vi "Engine - Copy & Script PPLTemplates (Inline-Async).vi"(7 "CD Name":string, 8 "error in (no error)":errorcluster, 9 "RT Driver VI Path":path, 10 "RT Driver Folder Path":path, 11 "CD Source Folder Path":path) -> (0 "error out":errorcluster)   [LabVIEW 2019, in "NIVS_Consolidated_CDW_MetaDataObj.lvclass"]
doc: "Via scripting, replace the tempate RTStateVariables control with the new type def across the async and RT driver VIs, and script the compiled settings property into the constants global"
uses:
  NIVS_Consolidated_CDW_MetaDataObj.lvclass
  Common.ctl
  <vilib>/Utility/traverseref.llb/TRef TravTarget.ctl
  CD Engine lvlib.ctl
  CD Shared lvlib.ctl
  Common.vi
  CD Engine lvlib.vi
  CD Shared lvlib.vi
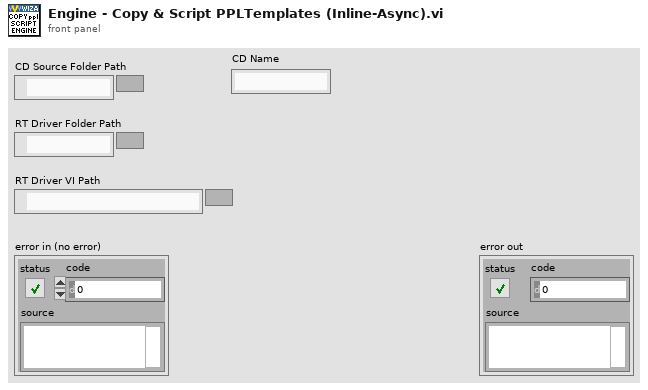
[diagram p1: front panel]
types:
  T1 = typedef "NIVS_Consolidated_CDW_MetaDataObj.lvclass/CD Engine lvlib.ctl" = enum16{"LibraryFileName", "LibraryFolderName", "Engine.FolderName", "Engine.Init.FolderName", "Engine.Run.FolderName", "Engine.Shutdown.FolderName", "Types.FolderName", "Engine.RT Driver VI.TemplatePath", "Engine.RT Driver VI.FileName", "Engine.RTStateVariables.Name", "Engine.RTStateVariables.Name.NoExtension", "Engine.Async.NameExtension", "Engine.Async.TemplateName", "Engine.PPL.Async.InitVSGlobals.Name"}
  T2 = typedef "NIVS_Consolidated_CDW_MetaDataObj.lvclass/CD Shared lvlib.ctl" = enum16{"LibraryFileName", "LibraryFolderName", "ConstantsVI.VIPathAndName", "Shared.FolderName", "Shared.Types.FolderName", "Shared.Constants.VIName", "Shared.Constants.VITemplateName", "Shared.Constants.VITemplatePathAndName", "Shared.CompiledSettings.RelativePath", "Shared.Constants.RelativePath", "Shared.CompiledSettings.Name", "Shared.CompiledSettings.Name.NoExtension", "Shared.CompiledSettings.ClusterName"}
  T3 = typedef "TRef TravTarget.ctl" = enum16{"FP", "BD", "Other"}
  T4 = typedef "NIVS_Consolidated_CDW_MetaDataObj.lvclass/Common.ctl" = enum16{"ProjectName", "TemplatesFolderName", "PPLTemplatesFolderName", "ProjectTemplatePathAndName", "ProjectPPLTemplatePathAndName", "TimingAndSyncFolderName", "CustomDeviceFolderName", "PathToTemplates", "PathToPPLTemplates", "PathToExplorerPPLTemplates", "PathToEnginePPLTemplates", "PathToConfigurationFile", "ProjectConfigurationName"}
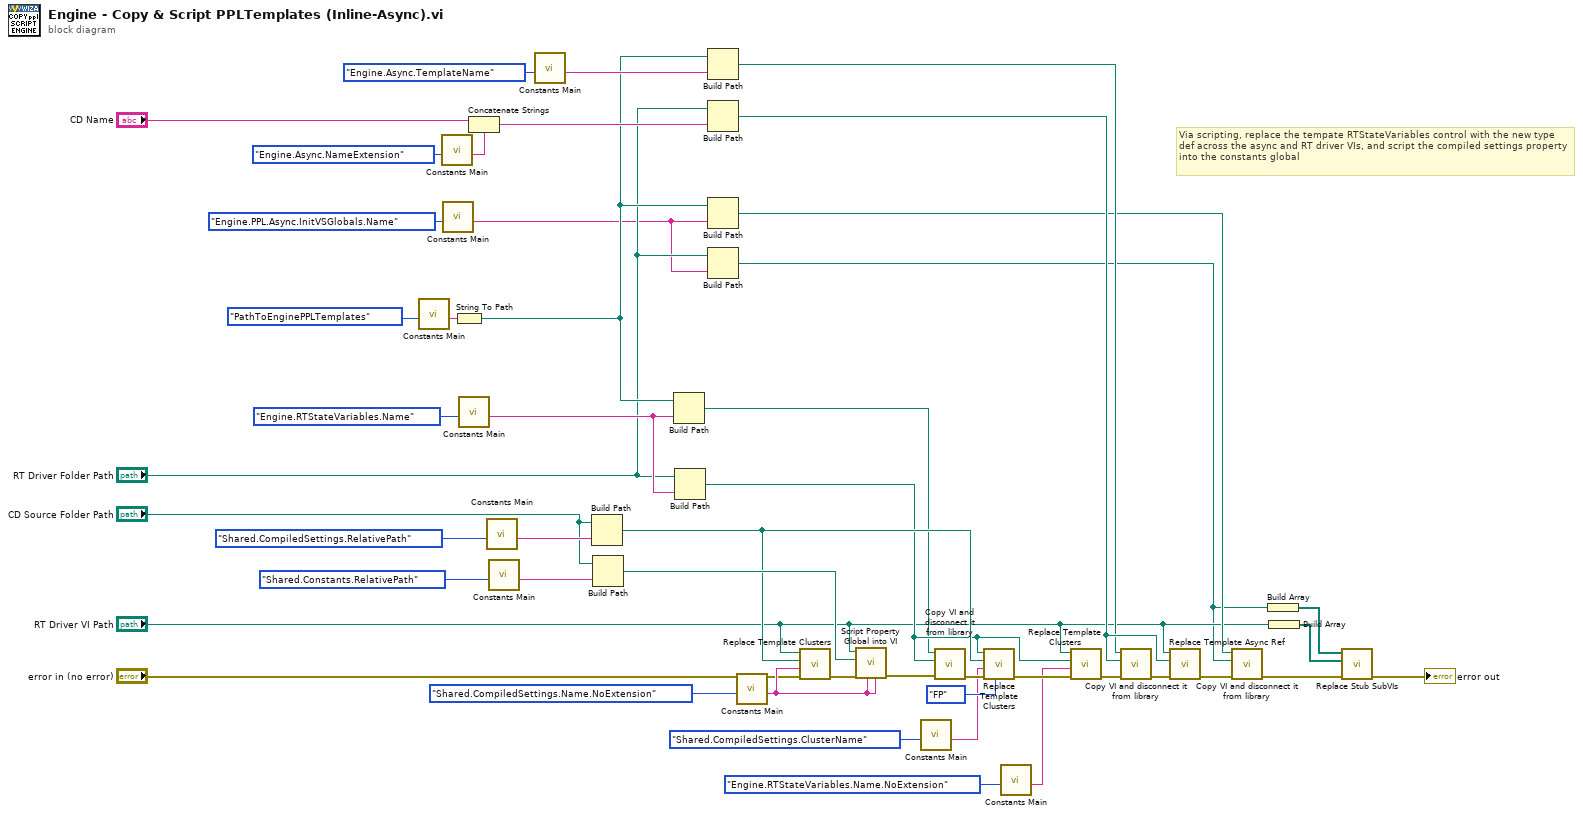
[diagram p0: block diagram]
diagram:
  # "Via scripting, replace the tempate RTStateVariables control with the new type def across the async and RT driver VIs, and script the compiled settings property into the constants global"
  n1 = call-poly "Constants Main.vi"("Action"=Common."PathToEnginePPLTemplates") -> ("Output"=w33:string)  [unwired: 10 in]
  n2 = call-poly "Constants Main.vi"("Action"=CD_Engine_lvlib."Engine.Async.NameExtension") -> ("Output"=w30:string)  [unwired: 10 in]
  n3 = call-poly "Constants Main.vi"("Action"=CD_Engine_lvlib."Engine.PPL.Async.InitVSGlobals.Name") -> ("Output"=w7:string)  [unwired: 10 in]
  n4 = String To Path(string=w33) -> (path=w10:path)
  n5 = call-poly "Constants Main.vi"("Action"=CD_Engine_lvlib."Engine.RTStateVariables.Name") -> ("Output"=w21:string)  [unwired: 10 in]
  n6 = Concatenate Strings("CD Name", w30) -> (w41:string)
  n7 = call-poly "Constants Main.vi"("Action"=CD_Shared_lvlib."Shared.CompiledSettings.RelativePath") -> ("Output"=w26:string)  [unwired: 10 in]
  n8 = call-poly "Constants Main.vi"("Action"=CD_Shared_lvlib."Shared.Constants.RelativePath") -> ("Output"=w24:string)  [unwired: 10 in]
  n9 = call-poly "Constants Main.vi"("Action"=CD_Engine_lvlib."Engine.Async.TemplateName") -> ("Output"=w28:string)  [unwired: 10 in]
  n10 = Build Path(base path="CD Source Folder Path", name or relative path=w26) -> (appended path=w46:path)
  n11 = Build Path(base path="CD Source Folder Path", name or relative path=w24) -> (appended path=w47:path)
  n12 = Build Path(base path=w10, name or relative path=w21) -> (appended path=w34:path)
  n13 = Build Path(base path="RT Driver Folder Path", name or relative path=w21) -> (appended path=w38:path)
  n14 = Build Path(base path=w10, name or relative path=w28) -> (appended path=w40:path)
  n15 = Build Path(base path="RT Driver Folder Path", name or relative path=w41) -> (appended path=w43:path)
  n16 = Build Path(base path=w10, name or relative path=w7) -> (appended path=w9:path)
  n17 = Build Path(base path="RT Driver Folder Path", name or relative path=w7) -> (appended path=w1:path)
  n18 = call-poly "Constants Main.vi"("Action"=CD_Shared_lvlib."Shared.CompiledSettings.Name.NoExtension") -> ("Output"=w19:string)  [unwired: 10 in]
  n19 = call "Replace Template Clusters.vi"("error in (no error)"="error in (no error)", "Control Name"=w19, "Path to Cluster to Replace"=w46, "Path to VI"="RT Driver VI Path") -> ("error out"=w44:errorcluster)  [unwired: 7 in]
  n20 = call "Script Property Global into VI.vi"("GlobalControlName"=w19, "StringConstantToReplace"=w19, "error in (no error)"=w44, "Path to Global"=w47, "Path to VI"="RT Driver VI Path") -> ("error out"=w45:errorcluster)  [unwired: 6 in]
  n21 = call-poly "Constants Main.vi"("Action"=CD_Shared_lvlib."Shared.CompiledSettings.ClusterName") -> ("Output"=w17:string)  [unwired: 10 in]
  n22 = call "Copy VI and disconnect it from library.vi"("error in (no error)"=w45, "VI Target Path"=w38, "VI Source Path"=w34) -> ("error out"=w35:errorcluster)  [unwired: 8 in]
  n23 = call "Replace Template Clusters.vi"("Traverse Target"=TRef_TravTarget."FP", "error in (no error)"=w35, "Control Name"=w17, "Path to Cluster to Replace"=w46, "Path to VI"=w38) -> ("error out"=w37:errorcluster)  [unwired: 6 in]
  n24 = call-poly "Constants Main.vi"("Action"=CD_Engine_lvlib."Engine.RTStateVariables.Name.NoExtension") -> ("Output"=w15:string)  [unwired: 10 in]
  n25 = call "Replace Template Clusters.vi"("error in (no error)"=w37, "Control Name"=w15, "Path to Cluster to Replace"=w38, "Path to VI"="RT Driver VI Path") -> ("error out"=w39:errorcluster)  [unwired: 7 in]
  n26 = call "Copy VI and disconnect it from library.vi"("error in (no error)"=w39, "VI Target Path"=w43, "VI Source Path"=w40) -> ("error out"=w42:errorcluster)  [unwired: 8 in]
  n27 = call "Replace Template Async Ref.vi"("error in (no error)"=w42, "Path to Desired Async VI"=w43, "Path to RT Driver VI"="RT Driver VI Path") -> ("error out"=w12:errorcluster)  [unwired: 8 in]
  n28 = call "Copy VI and disconnect it from library.vi"("error in (no error)"=w12, "VI Target Path"=w1, "VI Source Path"=w9) -> ("error out"=w6:errorcluster)  [unwired: 8 in]
  n29 = Build Array(w1) -> (w2:path[])
  n30 = Build Array("RT Driver VI Path") -> (w3:path[])
  n31 = call "Replace Stub SubVIs.vi"("error in"=w6, "VIs to Process"=w3, "subVIs to replace"=w2) -> ("error out"=→"error out":errorcluster)  [unwired: 8 in]
